vi "Done Glyph.vi"(8 "error in (no error)":errorcluster, 11 "glyph ref in":i64) -> (0 "error out":errorcluster)   [LabVIEW 2023, in "Freetype Drawer.lvlib"]
uses:
  Freetype Drawer.lvlib
  libfreetype.dll
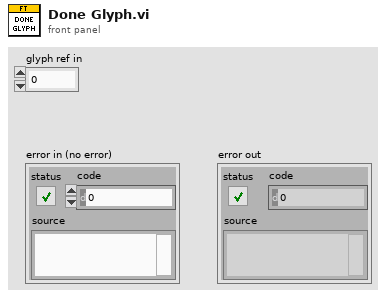
[diagram p1: front panel]
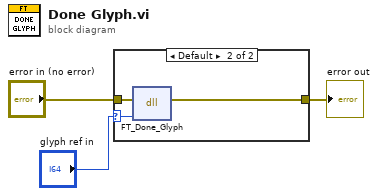
[diagram p0: block diagram]
diagram:
  n1 = case shown="Default" "glyph ref in" {
    selector: "glyph ref in" -> [_ w7]
    tunnel: [w4 w6] -> w2
    tunnel: "error in (no error)" -> [w4 w5]
    frame 0 {
    }
    frame Default {
      n2 = dll-call lib="E:/Labview/LV 2023/Libs/LV Symbol/Freetype Drawer/Wrappers/libfreetype.dll" fn="FT_Done_Glyph"(error in=w5, "glyph in"=w7) -> (error out=w6:errorcluster)  [unwired: 4 in, 1 out]
    }
  }
  "error out" <- w2
